vi "Step Mode - Configure Time Unit.vi"(8 "error in (no error)":errorcluster, 10 "Unit":u16(ring) items=["MILLISECOND", "SECOND", "MINUTE", "HOUR"], 11 "VISA resource name":refnum<visa-resource-name>) -> (0 "error out":errorcluster, 3 "VISA resource name out":refnum<visa-resource-name>)   [LabVIEW 2014, in "Associated Power Technologies 8500 Series.lvlib"]
doc: "Configure the time unit, including millisecond, second, minute or hour."
uses:
  <instrlib>/Associated Power Technologies 8500 Series/Associated Power Technologies 8500 Series.lvlib
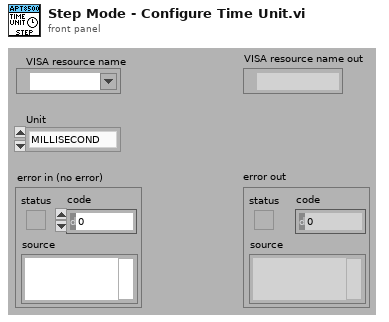
[diagram p1: front panel]
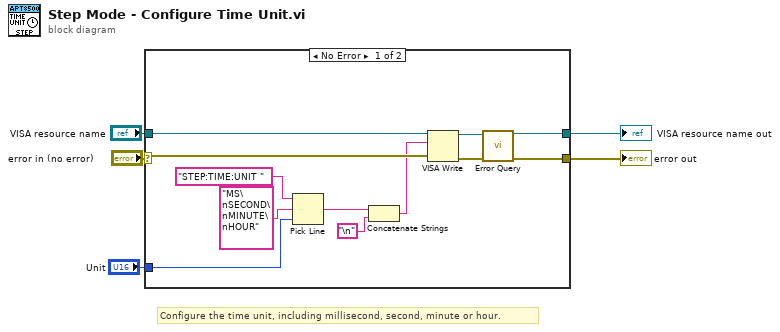
[diagram p0: block diagram]
diagram:
  # "Configure the time unit, including millisecond, second, minute or hour."
  n1 = case shown="No Error" "error in (no error)" {
    selector: "error in (no error)" -> [w16 w19]
    tunnel: "VISA resource name" -> [w17 w18]
    tunnel: [w15 w18] -> w5
    tunnel: [w14 w19] -> w4
    tunnel: "Unit" -> [w8 _]
    frame No Error {
      n2 = Pick Line(string ("")="STEP:TIME:UNIT ", multi-line string="MS\nSECOND\nMINUTE\nHOUR", line index=w8) -> (output string=w9:string)
      n3 = Concatenate Strings(w9, "\n") -> (w7:string)
      n4 = VISA Write(VISA resource name=w17, write buffer=w7, error in (no error)=w16) -> (VISA resource name out=w13:refnum<visa-resource-name>, error out=w12:errorcluster)  [unwired: 1 out]
      n5 = call <instrlib>:"Error Query.vi"("VISA resource name"=w13, "error in (no error)"=w12) -> ("VISA resource name out"=w15:refnum<visa-resource-name>, "error out"=w14:errorcluster)  [unwired: 10 in, 2 out]
    }
    frame Error {
    }
  }
  "error out" <- w4
  "VISA resource name out" <- w5
